vi "Variable list Stroker analog.vi"() -> (6 "Variant":variant, 10 "Array":T1[](array[typedef]) {"Default Scaling"."Offset" format="%.5f"; "Default Scaling"."Gain" format="%.5f"})   [LabVIEW 2011]
uses:
  Measurments Handling/Fixed Analog Channel Definition.ctl
  Measurments Handling/Units/Quantity enum.ctl
  Measurments Handling/Update frequensies.ctl
  Measurments Handling/Channel catagory Enum.ctl
  Measurments Handling/Scaling.ctl
  Variable List Stroker Analog.ctl
  <vilib>/Utility/VariantDataType/GetNumericInfo.vi
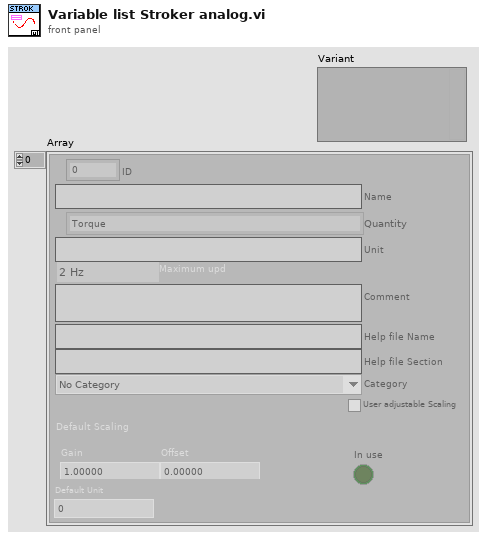
[diagram p1: front panel]
types:
  T1 = typedef "Fixed Analog Channel Definition.ctl" = cluster{"ID":u16, "Name":string, "Quantity":T2, "Unit":string, "Maximum upd":T3, "Comment":string, "Help file Name":string, "Help file Section ":string, "Category":T4, "User adjustable Scaling":bool, "Default Scaling":T5, "In use":bool, "Default Unit":i32}
  T2 = typedef "Quantity enum.ctl" = enum16{"Acceleration", "Angle", "Current", "Force", "Distance", "Pressure", "Resistance", "Rotational Speed", "Speed", "Temperature", "Tension", "Torque", "Voltage", "Weight"}
  T3 = typedef "Update frequensies.ctl" = enum16{"2 Hz", "1 Hz", "0.1 Hz"}
  T4 = typedef "Channel catagory Enum.ctl" = enum16{"No Category", "Power", "Temperature", "Pressure"}
  T5 = typedef "Scaling.ctl" = cluster{"Gain":dbl, "Offset":dbl}
  T6 = typedef "Variable List Stroker Analog.ctl" = enum16{"Tool max Temperature", "Solenoid Temp", "Tool supply Voltage", "Tool (Controller) Current", "Tool Acceleration X", "Tool Acceleration Y", "Tool Acceleration Z", "Controller Temp", "Tool Acceleration Sum", "Tool Inclination", "Tool Rotation", "Tool Stroke Extension", "Tool GP Sensor 1", "Tool GP Sensor 2", "Tool (Pressure 1) Temp", "Tool Pressure 1", "Tool (Pressure 2) Temp", "Tool Pressure 2", "Do not use (SIF)", "Do not use (SOF)", "Stroke Force", "PSU Temp", "Head Voltage", "PSU Main Voltage out", "PSU Main Current out", "Upper Tension Sub Temp", "Tool Upper Tension Sub", "Lower Tension Sub Temp", "Tool Lower Tension Sub"}
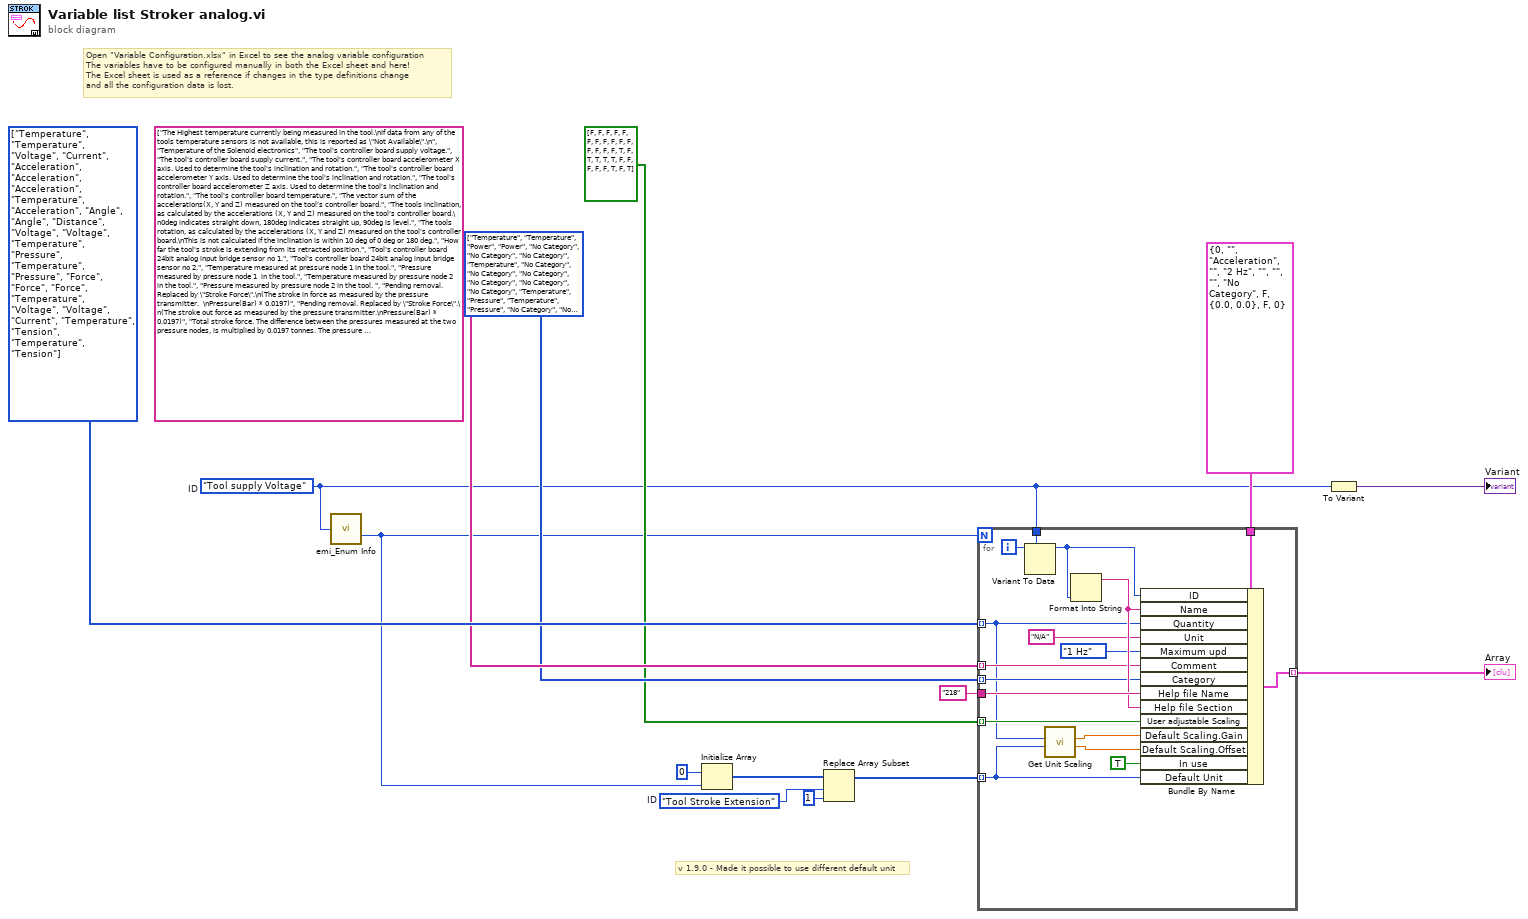
[diagram p0: block diagram]
diagram:
  w3 = Variable_List_Stroker_Analog."Tool Stroke Extension"  # ID
  w10 = T4[] [enum."Temperature", enum."Temperature", enum."Power", enum."Power", enum."No Category", enum."No Category", enum."No Category", enum."Temperature", enum."No Category", enum."No Category", enum."No Category", enum."No Category", enum."No Category", enum."No Category", enum."Temperature", enum."Pressure", enum."Temperature", enum."Pressure", enum."No Category", enum."No Category", enum."No Category", enum."No Category", enum."No Category", enum."No Category", enum."No Category", enum."Temperature", enum."No Category", enum."Temperature", enum."No Category"] items=["No Category", "Power", "Temperature", "Pressure"]
  w12 = T2[] [enum."Temperature", enum."Temperature", enum."Voltage", enum."Current", enum."Acceleration", enum."Acceleration", enum."Acceleration", enum."Temperature", enum."Acceleration", enum."Angle", enum."Angle", enum."Distance", enum."Voltage", enum."Voltage", enum."Temperature", enum."Pressure", enum."Temperature", enum."Pressure", enum."Force", enum."Force", enum."Force", enum."Temperature", enum."Voltage", enum."Voltage", enum."Current", enum."Temperature", enum."Tension", enum."Temperature", enum."Tension"] items=["Acceleration", "Angle", "Current", "Force", "Distance", "Pressure", "Resistance", "Rotational Speed", "Speed", "Temperature", "Tension", "Torque", "Voltage", "Weight"]
  w7 = Variable_List_Stroker_Analog."Tool supply Voltage"  # ID
  # "v 1.9.0 - Made it possible to use different default unit"
  # "Open \"Variable Configuration.xlsx\" in Excel to see the analog variable configuration\nThe variables have to be configured manually in both the Excel sheet and here!\nThe Excel sheet is used as a reference if changes in the type definitions change\nand all the configuration data is lost."
  n1 = call "emi_Enum Info.vi"("Enum"=w7) -> ("Numb Elements"=w6:i32)  [unwired: 11 in, 3 out]
  n2 = Initialize Array(0, w6) -> (w4:i32[])
  n3 = Replace Array Subset(array=w4, new element=1 ("new element/subarray"), index=w3) -> (w1:i32[])
  n4 = for {
    N: w6 -> [_]
    tunnel: "218" ("Help file Name") -> [w30]
    tunnel: [w32] -> w8 mode=indexing
    tunnel: T1 {"ID"=0, "Name"="", "Quantity"=enum."Acceleration", "Unit"="", "Maximum upd"=enum."2 Hz", "Comment"="", "Help file Name"="", "Help file Section "="", "Category"=enum."No Category", "User adjustable Scaling"=FALSE, "Default Scaling"={"Gain"=0.0, "Offset"=0.0}, "In use"=FALSE, "Default Unit"=0} ("Variable Defenition") -> [w31]
    tunnel: w12 -> [w20] mode=indexing
    tunnel: w7 -> [w28]
    tunnel: string[] ["The Highest temperature currently being measured in the tool.\nIf data from any of the tools temperature sensors is not available, this is reported as \"Not Available\".\n", "Temperature of the Solenoid electronics", "The tool's controller board supply voltage.", "The tool's controller board supply current.", "The tool's controller board accelerometer X axis. Used to determine the tool's inclination and rotation.", "The tool's controller board accelerometer Y axis. Used to determine the tool's inclination and rotation.", "The tool's controller board accelerometer Z axis. Used to determine the tool's inclination and rotation.", "The tool's controller board temperature.", "The vector sum of the accelerations(X, Y and Z) measured on the tool's controller board.", "The tools inclination, as calculated by the accelerations (X, Y and Z) measured on the tool's controller board.\n0deg indicates straight down, 180deg indicates straight up, 90deg is level.", "The tools rotation, as calculated by the accelerations (X, Y and Z) measured on the tool's controller board.\nThis is not calculated if the inclination is within 10 deg of 0 deg or 180 deg.", "How far the tool's stroke is extending from its retracted position.", "Tool's controller board 24bit analog input bridge sensor no 1.", "Tool's controller board 24bit analog input bridge sensor no 2.", "Temperature measured at pressure node 1 in the tool.", "Pressure measured by pressure node 1  in the tool.", "Temperature measured by pressure node 2  in the tool.", "Pressure measured by pressure node 2 in the tool. ", "Pending removal. Replaced by \"Stroke Force\".\n(The stroke in force as measured by the pressure transmitter.  \nPressure(Bar) * 0.0197)", "Pending removal. Replaced by \"Stroke Force\".\n(The stroke out force as measured by the pressure transmitter.\nPressure(Bar) * 0.0197)", "Total stroke force. The difference between the pressures measured at the two pressure nodes, is multiplied by 0.0197 tonnes. The pressure of Node 2 is subtracted from the pressure of Node 1.", "Temperature measured in PSU", "Input voltage of PSU", "Output voltage of PSU", "Output current of PSU", "Temperature measured at the upper tension sub node in the tool.", "Tension measured by the upper tension sub node in the tool.", "Temperature measured at the lower tension sub node in the tool.", "Tension measured by the lower tension sub node in the tool."] -> [w23] mode=indexing
    tunnel: w10 -> [w25] mode=indexing
    tunnel: bool[] [FALSE, FALSE, FALSE, FALSE, FALSE, FALSE, FALSE, FALSE, FALSE, FALSE, FALSE, FALSE, FALSE, FALSE, FALSE, TRUE, FALSE, TRUE, TRUE, TRUE, TRUE, FALSE, FALSE, FALSE, FALSE, FALSE, TRUE, FALSE, TRUE] -> [w24] mode=indexing
    tunnel: w1 -> [w16] mode=indexing
    i -> [w29]
    n5 = Variant To Data(type=w28, Variant=w29) -> (data=w27:T6)  [unwired: 1 in, 1 out]
    n6 = call "Get Unit Scaling.vi"("Unit Index"=w16, "Quantity"=w20) -> ("Offset"=w17:dbl, "Gain"=w18:dbl)  [unwired: 7 in, 1 out]
    n7 = Format Into String(w27) -> (resulting string=w26:string)  [unwired: 3 in, 1 out]
    n8 = Bundle By Name(cluster=w31, "ID"=w27, "Name"=w26, "Quantity"=w20, "Unit"="N/A", "Maximum upd"=Update_frequensies."1 Hz", "Comment"=w23, "Category"=w25, "Help file Name"=w30, "Help file Section"=w26, "User adjustable Scaling"=w24, "Default Scaling.Gain"=w18, "Default Scaling.Offset"=w17, "In use"=TRUE, "Default Unit"=w16) -> (w32:T1)
  }
  "Array" <- w8
  n9 = To Variant(anything=w7) -> (Variant=→"Variant":variant)
